vi "NI VeriStand - Search for All Items by Name.vi"(8 "error in":errorcluster, 10 "Item Name":string, 11 "Section Ref in":T1 format="%.0x") -> (0 "error out":errorcluster, 2 "Item Refs":T1[](array[typedef]) format="%.0x", 3 "Section Ref out":T1 format="%.0x", 4 "Found":bool)   [LabVIEW 2020, in "Custom Device Utility Library.lvlib"]
doc: "Searches a custom device section for the item(s) you specify. You can search for one or multiple items by name, GUID, or property name and value. You must manually select the polymorphic instance to use."
uses:
  <vilib>/NI VeriStand/Custom Device Tools/Custom Device Utility Library/Custom Device Utility Library.lvlib
  <vilib>/NI VeriStand/Custom Device API/Custom Device Item Ref.ctl
  <vilib>/NI VeriStand/Custom Device API/Custom Device API.lvlib
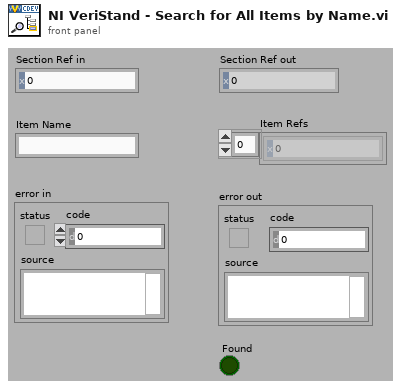
[diagram p1: front panel]
types:
  T1 = typedef "Custom Device API.lvlib/Custom Device Item Ref.ctl" = u64
  T2 = typedef "Custom Device API.lvlib/Custom Device Item Info.ctl" = cluster{"Name":string, "Is Channel":bool, "GUID":string, "Is Waveform":bool}
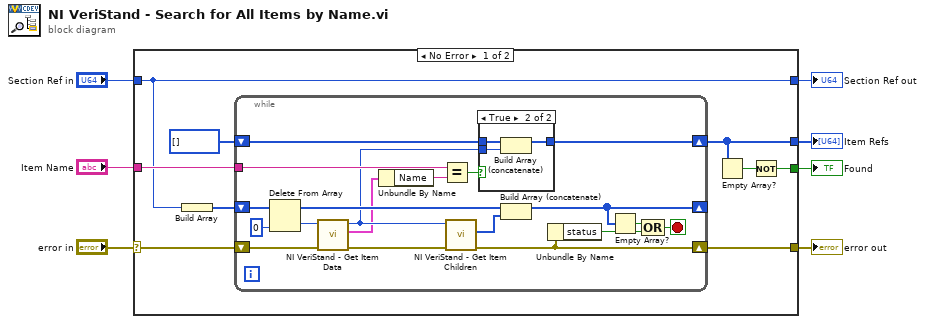
[diagram p0: block diagram]
diagram:
  n1 = case shown="No Error" "error in" {
    selector: "error in" -> [w9 w41]
    tunnel: "Section Ref in" -> [w8 w40]
    tunnel: "Item Name" -> [w15 _]
    tunnel: [w14 w41] -> w5
    tunnel: [w12 _] -> w4
    tunnel: [w10 _] -> w3
    tunnel: [w8 w40] -> w1
    frame No Error {
      n2 = Build Array(w8) -> (w16:T1[])
      n3 = while {
        shift-right: [w35] -> w14
        shift-left: w9 -> [w33]
        shift-right: [w26] -> _
        shift-left: w16 -> [w32]
        tunnel: w15 -> [w29]
        shift-right: [w20] -> w12
        shift-left: T1[] [] ("appended array") -> [w21]
        stop <- w23 stop-if-true
        n4 = Delete From Array(array=w32, index=0) -> (deleted portion=w30:T1, array with subset deleted=w28:T1[])  [unwired: 1 in]
        n5 = call <vilib>:"NI VeriStand - Get Item Data.vi"("error in (no error)"=w33, "Item Ref in"=w30) -> ("error out"=w34:errorcluster, "Item Info"=w18:T2, "Item Ref out"=w19:T1)  [unwired: 7 out]
        n6 = Unbundle By Name(w18) -> ("Name"=w17:string)
        n7 = Equal?(x=w29, y=w17) -> (x = y?=w22:bool)
        n8 = call <vilib>:"NI VeriStand - Get Item Children.vi"("error in (no error)"=w34, "Item Ref in"=w19) -> ("error out"=w35:errorcluster, "Child Refs"=w27:T1[])  [unwired: 8 out]
        n9 = case shown="True" w22 {
          tunnel: w21 -> [w36 w39]
          tunnel: [w36 w38] -> w20
          tunnel: w19 -> [_ w37]
          frame False {
          }
          frame True {
            n10 = Build Array (concatenate)(w39, w37) -> (w38:T1[])
          }
        }
        n11 = Build Array (concatenate)(w28, w27) -> (w26:T1[])
        n12 = Unbundle By Name(w35) -> ("status"=w25:bool)
        n13 = Empty Array?(array=w26) -> (empty?=w24:bool)
        n14 = Compound Arithmetic op=OR(w24, w25) -> (w23:bool)
      }
      n15 = Empty Array?(array=w12) -> (empty?=w11:bool)
      n16 = Not(x=w11) -> (.not. x?=w10:bool)
    }
    frame Error {
    }
  }
  "Found" <- w3
  "error out" <- w5
  "Section Ref out" <- w1
  "Item Refs" <- w4
